vi "runReady.vi"(4 "FullRun? in":bool, 6 "Fault?":bool, 7 "Time in":dbl, 8 "error in (no error)":errorcluster, 9 "Actuators in":T2, 10 "State in":T1, 11 "FullRun in":refnum<class "FullRun.lvclass">) -> (0 "error out":errorcluster, 1 "Actuators out":T2, 2 "State out":T1, 3 "FullRun out":refnum<class "FullRun.lvclass">, 5 "FullRun? out":bool)   [LabVIEW 2018, in "ControlLibrary.lvlib" / "FullRun.lvclass"]
uses:
  FullRun.lvclass
  TypeDef_DigitalOuts.ctl
  TypeDef_ControlState.ctl
  RunTypeClass/RunType.lvclass
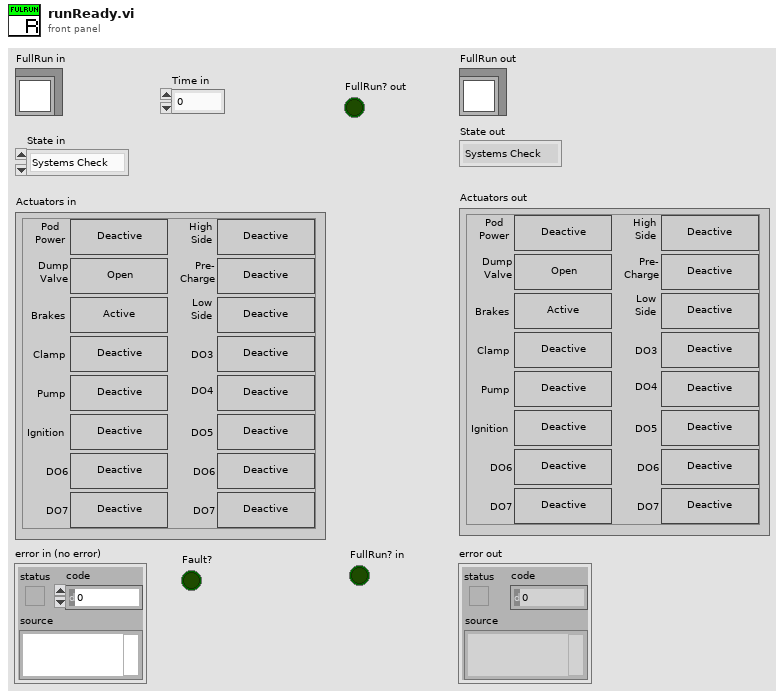
[diagram p1: front panel]
types:
  T1 = typedef "TypeDef_ControlState.ctl" = enum16{"Systems Check", "Idle", "Ready", "Pushing", "Coast", "Braking", "Fault", "Shutdown", "Service", "Precharge", "Blank"}
  T2 = typedef "TypeDef_DigitalOuts.ctl" = cluster{"Pod Power":bool, "Dump Valve":bool, "Brakes":bool, "Clamp":bool, "Pump":bool, "Ignition":bool, "DO6":bool, "DO7":bool, "HighSide":bool, "Precharge":bool, "LowSide":bool, "DO3":bool, "DO4":bool, "DO5":bool, "DO62":bool, "DO72":bool}
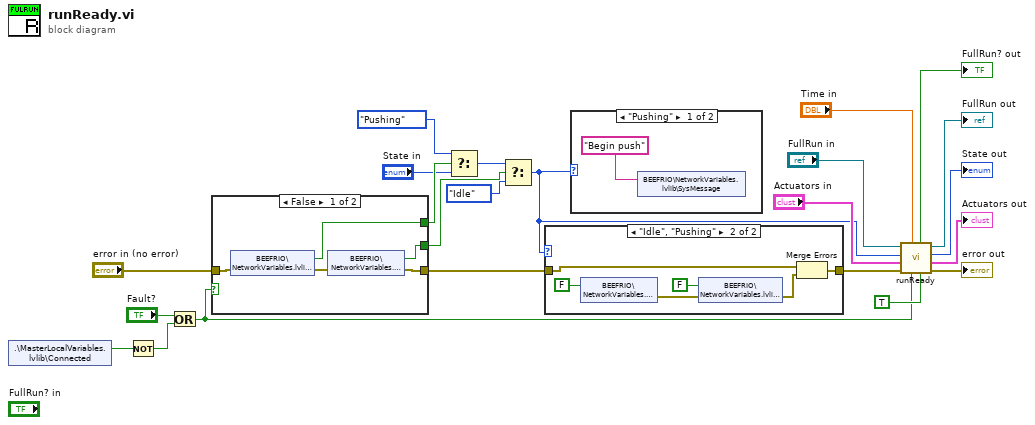
[diagram p0: block diagram]
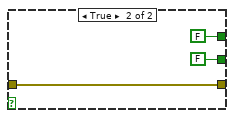
[diagram p3: hidden frame]
diagram:
  n1 = shared-variable ".\\MasterLocalVariables.lvlib\\Connected"() -> (w4:bool)  [unwired: 1 in, 1 out]
  n2 = Not(x=w4) -> (.not. x?=w2:bool)
  n3 = Or(x="Fault?", y=w2) -> (x .or. y?=w3:bool)
  n4 = case shown="False" w3 {
    tunnel: [w27 FALSE ("Boolean")] -> w15
    tunnel: [w24 FALSE ("Boolean")] -> w12
    tunnel: "error in (no error)" -> [w26 w30]
    tunnel: [w25 w30] -> w11
    frame False {
      n5 = shared-variable "BEEFRIO\\NetworkVariables.lvlib\\Launch"(error in=w26) -> (w27:bool, error out=w28:errorcluster)
      n6 = shared-variable "BEEFRIO\\NetworkVariables.lvlib\\Ready"(error in=w28) -> (w24:bool, error out=w25:errorcluster)
    }
    frame True {
    }
  }
  n7 = Select(t=TypeDef_ControlState."Pushing" ("Next State"), s=w15, f="State in") -> (s? t:f=w10:T1)
  n8 = Select(t=w10, s=w12, f=TypeDef_ControlState."Idle" ("Next State")) -> (s? t:f=w1:T1)
  n9 = case shown="\"Idle\", \"Pushing\"" w1 {
    tunnel: w11 -> [w32 w33]
    tunnel: [w32 w35] -> w6
    frame Default {
    }
    frame "Idle", "Pushing" {
      n10 = shared-variable "BEEFRIO\\NetworkVariables.lvlib\\Ready"(FALSE ("Ready")) -> (error out=w37:errorcluster)  [unwired: 1 in]
      n11 = shared-variable "BEEFRIO\\NetworkVariables.lvlib\\Launch"(FALSE ("Launch"), error in=w37) -> (error out=w34:errorcluster)
      n12 = Merge Errors(w33, w34) -> (w35:errorcluster)
    }
  }
  n13 = case shown="\"Pushing\"" w1 {
    frame "Pushing" {
      n14 = shared-variable "BEEFRIO\\NetworkVariables.lvlib\\SysMessage"("Begin push") -> ()  [unwired: 1 in, 1 out]
    }
    frame Default {
    }
  }
  n15 = call-parent "runReady.vi"("FullRun? in"=TRUE, "Fault?"=w3, "Time in"="Time in", "error in (no error)"=w6, "Actuators in"="Actuators in", "State in"=w1, "RunType in"="FullRun in") -> ("error out"=→"error out":errorcluster, "Actuators out"=→"Actuators out":T2, "State out"=→"State out":T1, "RunType out"=→"FullRun out":refnum<class "FullRun.lvclass">, "FullRun? out"=→"FullRun? out":bool)
